vi "例程45-子面板.vi"() -> ()   [LabVIEW 2016]
panel:
  in  "子程序面板":bool
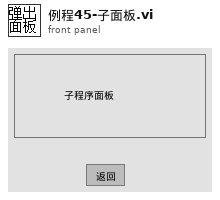
[diagram p1: front panel]
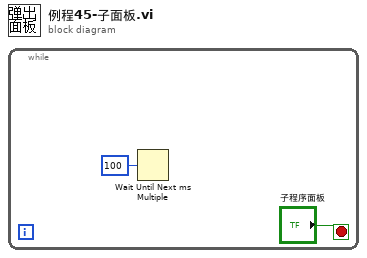
[diagram p0: block diagram]
diagram:
  n1 = while {
    stop <- "子程序面板" stop-if-true
    n2 = Wait Until Next ms Multiple(millisecond multiple=u32 100 ("毫秒倍数")) -> ()  [unwired: 1 out]
  }
